vi "com finder single cycle.vi"(9 "end of volume":bool, 10 "sampling values in":T2, 11 "current location":T1) -> (2 "com updated":bool, 3 "center of mass":cluster{"x avg":i16, "y avg":i16, "z avg":i16})   [LabVIEW 2010]
uses:
  common_typedefs/channels_cluster.ctl
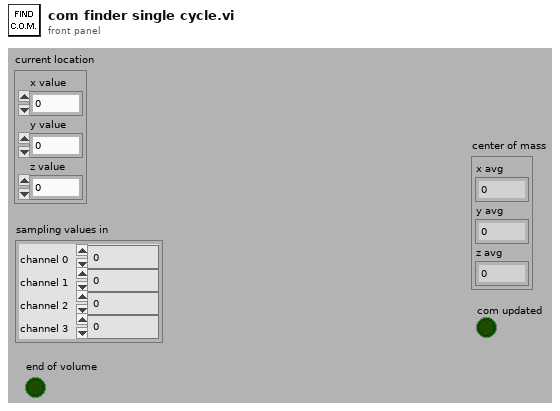
[diagram p1: front panel]
types:
  T1 = cluster{"x value":i16, "y value":i16, "z value":i16}
  T2 = typedef "channels_cluster.ctl" = cluster{"channel 0":u32, "channel 1":u32, "channel 2":u32, "channel 3":u32}
  T3 = cluster{"total photon count":u32, "x weighted sum":i32, "y weighted sum":i32, "z weighted sum":i32}
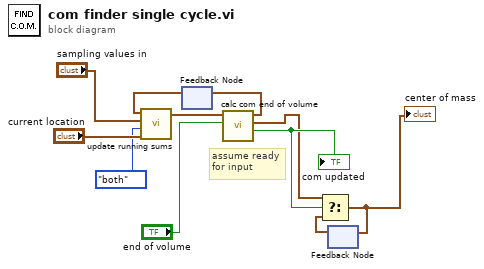
[diagram p0: block diagram]
diagram:
  # "assume ready\nfor input"
  n1 = feedback #1() -> (w7:T3)  [unwired: 1 in]
  n2 = call "update running sums.vi"("current location"="current location", "integration channels"=enum16{"channel 0", "channel 1", "both"}."both", "sampling values in"="sampling values in", "running sums in"=w7) -> ("running sums out"=w9:T3)  [unwired: 7 in]
  n3 = call "calc com end of volume.vi"("end of volume"="end of volume", "running sums in"=w9) -> ("output valid"=w5:bool, "center of mass"=w4:cluster{"x avg":i16, "y avg":i16, "z avg":i16}, "running sums out"=w8:T3)  [unwired: 6 in, 1 out]
  "com updated" <- w5
  n4 = feedback-in #1(w8) -> ()
  n5 = feedback #2() -> (w3:cluster{"x avg":i16, "y avg":i16, "z avg":i16})  [unwired: 1 in]
  n6 = Select(t=w4, s=w5, f=w3) -> (s? t:f=w2:cluster{"x avg":i16, "y avg":i16, "z avg":i16})
  "center of mass" <- w2
  n7 = feedback-in #2(w2) -> ()
